vi "ToDo.vi"   [LabVIEW 2014]
uses:
  MongoDB.Collection.lvclass
  C:/MongoData/Drivers/mongo-csharp-driver-2.0.0-beta4/mongo-csharp-driver-2.0.0-beta4/src/MongoDB.Driver.Legacy/bin/Release/MongoDB.Driver.Legacy.dll
  MongoData/Drivers/mongo-csharp-driver-2.0.0-beta4/mongo-csharp-driver-2.0.0-beta4/src/MongoDB.Driver.Legacy/bin/Release/MongoDB.Driver.Legacy.dll
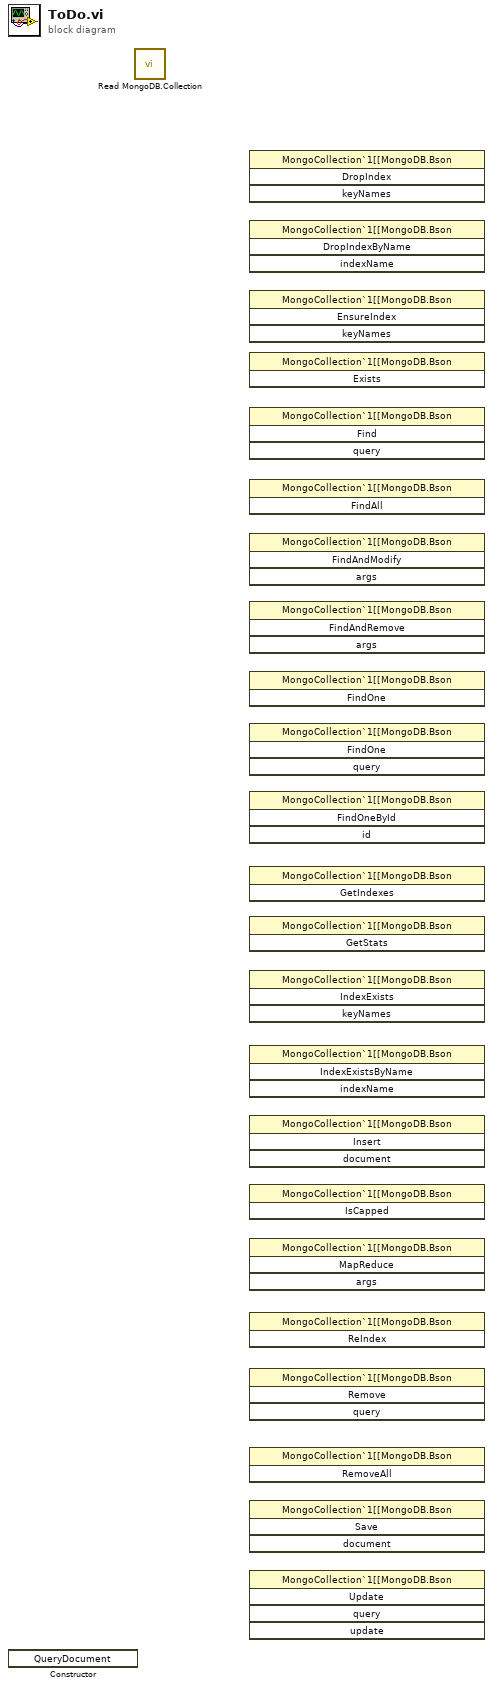
[diagram p0: block diagram]
diagram:
  n1 = constructor class="QueryDocument"() -> ()  [unwired: 3 in, 3 out]
  n2 = call "Read MongoDB.Collection.vi"() -> ()  [unwired: 9 in, 3 out]
  n3 = invoke class="MongoCollection`1[[MongoDB.Bson" method="DropIndex"() -> ()  [unwired: 4 in, 4 out]
  n4 = invoke class="MongoCollection`1[[MongoDB.Bson" method="DropIndexByName"() -> ()  [unwired: 4 in, 4 out]
  n5 = invoke class="MongoCollection`1[[MongoDB.Bson" method="EnsureIndex"() -> ()  [unwired: 4 in, 4 out]
  n6 = invoke class="MongoCollection`1[[MongoDB.Bson" method="Exists"() -> ()  [unwired: 3 in, 3 out]
  n7 = invoke class="MongoCollection`1[[MongoDB.Bson" method="Find"() -> ()  [unwired: 4 in, 4 out]
  n8 = invoke class="MongoCollection`1[[MongoDB.Bson" method="FindAll"() -> ()  [unwired: 3 in, 3 out]
  n9 = invoke class="MongoCollection`1[[MongoDB.Bson" method="FindAndModify"() -> ()  [unwired: 4 in, 4 out]
  n10 = invoke class="MongoCollection`1[[MongoDB.Bson" method="FindAndRemove"() -> ()  [unwired: 4 in, 4 out]
  n11 = invoke class="MongoCollection`1[[MongoDB.Bson" method="FindOne"() -> ()  [unwired: 3 in, 3 out]
  n12 = invoke class="MongoCollection`1[[MongoDB.Bson" method="FindOne"() -> ()  [unwired: 4 in, 4 out]
  n13 = invoke class="MongoCollection`1[[MongoDB.Bson" method="FindOneById"() -> ()  [unwired: 4 in, 4 out]
  n14 = invoke class="MongoCollection`1[[MongoDB.Bson" method="GetIndexes"() -> ()  [unwired: 3 in, 3 out]
  n15 = invoke class="MongoCollection`1[[MongoDB.Bson" method="GetStats"() -> ()  [unwired: 3 in, 3 out]
  n16 = invoke class="MongoCollection`1[[MongoDB.Bson" method="IndexExists"() -> ()  [unwired: 4 in, 4 out]
  n17 = invoke class="MongoCollection`1[[MongoDB.Bson" method="IndexExistsByName"() -> ()  [unwired: 4 in, 4 out]
  n18 = invoke class="MongoCollection`1[[MongoDB.Bson" method="Insert"() -> ()  [unwired: 4 in, 4 out]
  n19 = invoke class="MongoCollection`1[[MongoDB.Bson" method="IsCapped"() -> ()  [unwired: 3 in, 3 out]
  n20 = invoke class="MongoCollection`1[[MongoDB.Bson" method="MapReduce"() -> ()  [unwired: 4 in, 4 out]
  n21 = invoke class="MongoCollection`1[[MongoDB.Bson" method="ReIndex"() -> ()  [unwired: 3 in, 3 out]
  n22 = invoke class="MongoCollection`1[[MongoDB.Bson" method="Remove"() -> ()  [unwired: 4 in, 4 out]
  n23 = invoke class="MongoCollection`1[[MongoDB.Bson" method="RemoveAll"() -> ()  [unwired: 3 in, 3 out]
  n24 = invoke class="MongoCollection`1[[MongoDB.Bson" method="Save"() -> ()  [unwired: 4 in, 4 out]
  n25 = invoke class="MongoCollection`1[[MongoDB.Bson" method="Update"() -> ()  [unwired: 5 in, 5 out]
